vi "Test Variant to JSON 2.vi"() -> ()   [LabVIEW 2011]
uses:
  JSON Array/JSON Array.lvclass
  JSON Value/JSON Value.lvclass
  Variant JSON.lvlib
panel:
  in  "Test Cluster (convert to array)":T1={"T2"="test2", "T1"=456.789, "Nest"={"Enum"=enum."AAA", "NestNest"={"A"="Hi", "Extended"=2.0, "C"=1}}, "Test Array"=[456.789, 2.0, 3.0], "Boolean"=FALSE, "Time Stamp"=timestamp(0 s since 1904-01-01)} {"T1" format="%#_24g"}
  out "JSON String":string
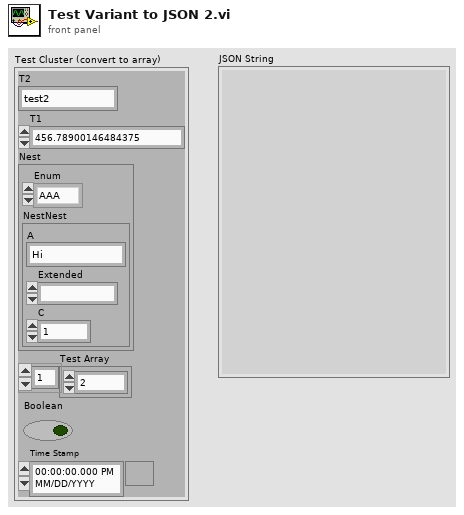
[diagram p1: front panel]
types:
  T1 = cluster{"T2":string, "T1":sgl, "Nest":cluster{"Enum":enum16{"AAA", "BBB", "CCC"}, "NestNest":cluster{"A":string, "Extended":ext, "C":i16}}, "Test Array":dbl[], "Boolean":bool, "Time Stamp":timestamp}
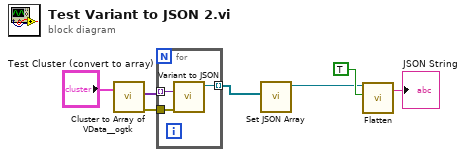
[diagram p0: block diagram]
diagram:
  n1 = call <userlib>:"Cluster to Array of VData__ogtk.vi"("Cluster"="Test Cluster (convert to array)") -> ("error out"=w5:errorcluster, "Array of VData"=w3:variant[])  [unwired: 9 in]
  n2 = for {
    tunnel: [w10] -> w2 mode=indexing
    tunnel: w5 -> [w9]
    tunnel: w3 -> [w8] mode=indexing
    n3 = call "Variant to JSON.vi"("error in (no error)"=w9, "Variant"=w8) -> ("JSON Value out"=w10:refnum<class "JSON Value.lvclass">)  [unwired: 8 in, 1 out]
  }
  n4 = call "Set JSON Array.vi"("Array"=w2) -> ("JSON Array out"=w1:refnum<class "JSON Array.lvclass">)  [unwired: 9 in, 1 out]
  n5 = call-dynamic "Flatten.vi"("Pretty Print?"=TRUE, "JSON Array in"=w1) -> ("String"=→"JSON String":string)  [unwired: 8 in, 1 out]
